vi "read_version.vi"() -> ()   [LabVIEW 2020]
uses:
  <vilib>/Automotive Diagnostic Command Set/Diagnostic Transport.llb/Transport Protocol Selector.ctl
  <vilib>/Automotive Diagnostic Command Set/Diagnostic Transport.llb/Property ID.ctl
  <vilib>/addons/Automotive Diagnostic Command Set/NI_Automotive Diagnostic Command Set.lvlib
panel:
  out "Response":u8[](array[numeric]) format="%.0x"
  out "CAN_log":string[][](table)
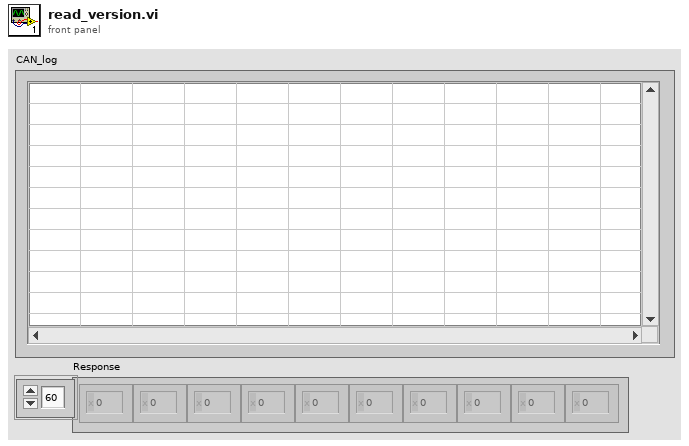
[diagram p1: front panel]
types:
  T1 = typedef "NI_Automotive Diagnostic Command Set.lvlib/Transport Protocol Selector.ctl" = enum16{"ISO TP - Normal Mode", "ISO TP - Mixed Mode", "VW TP 2.0", "Diagnostics on IP", "ISO TP LIN"}
  T2 = typedef "NI_Automotive Diagnostic Command Set.lvlib/Diag Reference.ctl" = cluster{"Diag CAN Handle":u32, "Transport Protocol":T1, "Receive Address Extension":u8, "Transmit Address Extension":u8, "Receive CAN Id":u32, "Transmit CAN Id":u32, "Log Frames ?":bool, "My TP Address":u8, "Other TP Address":u8, "T1":u16, "T2":u16, "T3":u16, "T4":u16, "Tx SN":u8, "Block Size":u8, "Rx SN":u8, "VW TP Initialized?":bool, "Tx block no":u8, "baud rate":u64, "Interface":string, "Channel Diag CAN Handle":u32, "UDP Connection ID":refnum<k16>, "TCP Connection ID":refnum<k5>, "Target IP Addr":u32, "Source Address":u16, "Target Address":u16, "Send Header NACK?":bool, "DLL Handle":u32, "NAD":u8, "Time Stamp read first":dbl, "Time Stamp read last":dbl, "Time Stamp write first":dbl, "Time Stamp write last":dbl, "Time Stamp write":dbl, "Time Stamp read":dbl, " I/O Mode":u32, "FD Baudrate":u64, "TX_DL":u16, "RX_DL":u16, "DoIP Protocol Version":T3, " Selected I/O Mode":u32, "TesterPresent Counter":u32, "TesterPresent Limit":u32, "TesterPresent Tick[ms]":i32, "TesterPresent RequireResponse?":bool, "TesterPresent Stored Ref?":bool, "TesterPresent Message":u8[], "TesterPresent Task Handle":i32, "TesterPresent Semaphore":T4, "Response Plausibility Check":u32, "Default Version?":bool, "Diagostic Globals":T5, "Session-based Properties?":bool}
  T3 = typedef "NI_Automotive Diagnostic Command Set.lvlib/DoIP Protocol Version.ctl" = u8
  T4 = typedef "Semaphore RefNum" = refnum<k1>
  T5 = typedef "NI_Automotive Diagnostic Command Set.lvlib/Diag Globals.ctl" = cluster{"Timeout FC (Bs)":u32, "Timeout CF (Cr)":u32, "Timeout Diag Command":u32, "Receive Block Size (BS)":u8, "Wait Time CF (STmin)":u8, "Max Waits (N_WFTmax)":u8, "Waits to Send (N_WAIT)":i32, "Time between Waits (TW)":u32, "Fill CAN Frames?":bool, "Fill Byte":u32, "Invalid Response as Error?":bool, "Max RspPending Count":u32, "VWTP Command Timeout":u32, "Transport Protocol":T1, "Diag CAN Handle":u32, "DLL Handle":u32, "Timeout RspPending":u32}
  T6 = typedef "NI_Automotive Diagnostic Command Set.lvlib/Property ID.ctl" = enum16{"Timeout Diag Command", "Timeout FC (Bs)", "Timeout CF (Cr)", "Receive Block Size (BS)", "Wait Time CF (STmin)", "Max Wait Frames (N_WFTmax)", "Wait Frames to Send (N_WAIT)", "Time between Waits (T_W)", "Fill CAN Frames", "Fill Byte", "Invalid Response as Error", "Max RspPending Count", "VWTP Command Timeout", "STmin", "P2min", "Termination", "Timeout RspPending", "LIN Sleep", "Actual CAN IO Mode", "Response Plausibility Check", "Session-based Properties"}
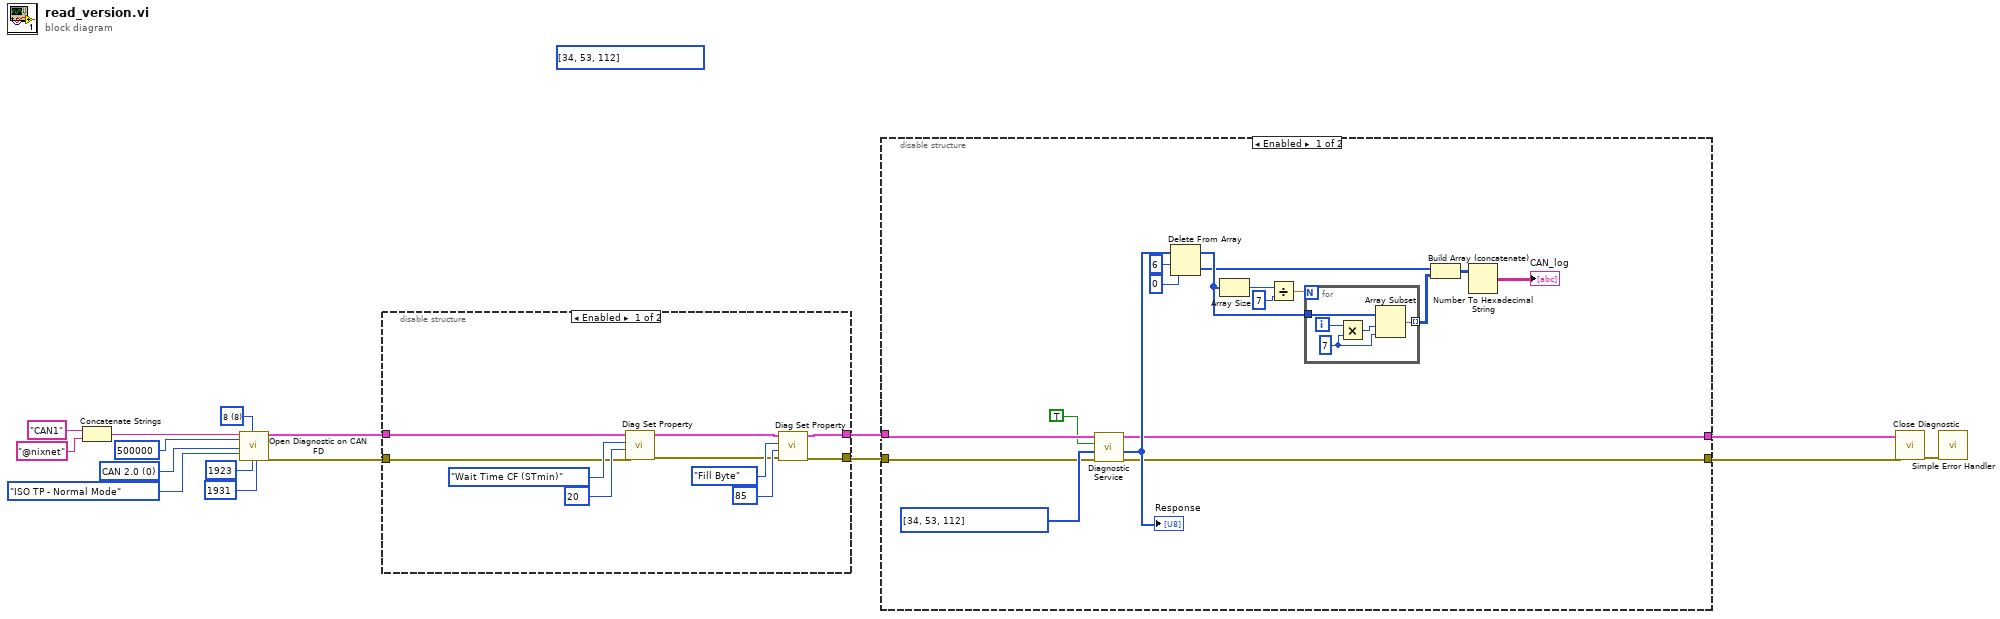
[diagram p0: block diagram]
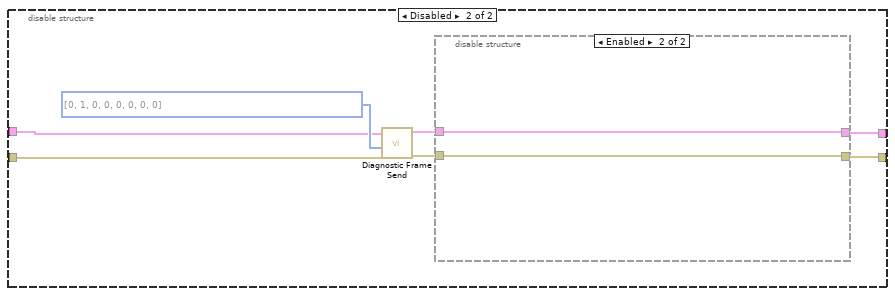
[diagram p3: hidden frame]
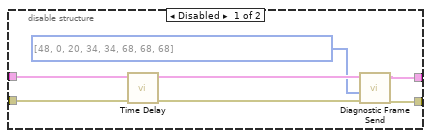
[diagram p4: hidden frame]
diagram:
  (unwired) u8[] [34, 53, 112] ("Request")
  w12 = u16 8 items=["8"=8, "12"=12, "16"=16, "20"=20, "24"=24, "32"=32, "48"=48, "64"=64] ("Max DLC")
  w14 = u32 0 items=["CAN 2.0", "CAN FD", "CAN FD+BRS", "ECU Determined"] ("IO Mode")
  n1 = Concatenate Strings("CAN1" ("Name"), "@nixnet") -> (w16:string)
  n2 = call <vilib>:"Open Diagnostic on CAN FD.vi"("CAN Interface"=w16, "Baud Rate"=u64 500000, "IO Mode"=w14, "Transport Protocol"=Transport_Protocol_Selector."ISO TP - Normal Mode", "Max DLC"=w12, "Transmit ID"=u32 1923, "Receive ID"=u32 1931) -> ("diag ref out"=w2:T2, "error out"=w1:errorcluster)  [unwired: 11 in]
  n3 = disable-structure shown="Enabled" {
    disable-tunnel: [w25 w28] -> w4
    disable-tunnel: [w24 w27] -> w3
    disable-tunnel: w2 -> [w20 w28]
    disable-tunnel: w1 -> [w18 w27]
    frame Enabled {
      n4 = call <vilib>:"Diag Set Property.vi"("error in (no error)"=w18, "property value"=u32 20, "property ID"=Property_ID."Wait Time CF (STmin)", "diag ref in"=w20) -> ("error out"=w17:errorcluster, "diag ref out"=w19:T2)  [unwired: 6 in]
      n5 = call <vilib>:"Diag Set Property.vi"("error in (no error)"=w17, "property value"=u32 85, "property ID"=Property_ID."Fill Byte", "diag ref in"=w19) -> ("error out"=w24:errorcluster, "diag ref out"=w25:T2)  [unwired: 6 in]
    }
    frame Disabled {
    }
  }
  n6 = disable-structure shown="Enabled" {
    disable-tunnel: w4 -> [w31 w52]
    disable-tunnel: w3 -> [w30 w51]
    disable-tunnel: [w34 w55] -> w6
    disable-tunnel: [w33 w54] -> w5
    frame Enabled {
      n7 = call <vilib>:"Diagnostic Service.vi"("error in (no error)"=w30, "data in"=u8[] [34, 53, 112] ("Request"), "require response?"=TRUE, "diag ref in"=w31) -> ("error out"=w33:errorcluster, "data out"=w45:u8[], "diag ref out"=w34:T2)  [unwired: 5 out]
      "Response" <- w45
      n8 = Delete From Array(array=w45, length=6, index=0) -> (deleted portion=w36:u8[], array with subset deleted=w39:u8[])
      n9 = Array Size(array=w39) -> (size(s)=w42:i32)
      n10 = Divide(x=w42, y=7) -> (x/y=w40:dbl)
      n11 = for {
        N: w40 -> [_]
        tunnel: w39 -> [w50]
        tunnel: [w46] -> w38 mode=indexing
        i -> [w48]
        w49 = 7 ("length")
        n12 = Multiply(x=w48, y=w49) -> (x*y=w47:i32)
        n13 = Array Subset(array=w50, index=w47, length=w49) -> (w46:u8[])
      }
      n14 = Build Array (concatenate)(w36, w38) -> (w37:u8[][])
      n15 = Number To Hexadecimal String(2:w37) -> (0:→"CAN_log":string[][])  [unwired: 1 in]
    }
    frame Disabled {
      n16 = call <vilib>:"Diagnostic Frame Send.vi"("error in (no error)"=w51, "data in"=u8[] [0, 1, 0, 0, 0, 0, 0, 0] ("Request"), "diag ref in"=w52) -> ("error out"=w57:errorcluster, "diag ref out"=w56:T2)  [unwired: 7 in]
      n17 = disable-structure shown="Enabled" {
        disable-tunnel: w57 -> [w63 w64]
        disable-tunnel: w56 -> [w62 w65]
        disable-tunnel: [w60 w65] -> w55
        disable-tunnel: [w59 w64] -> w54
        frame Disabled {
          n18 = call "Time Delay"("error in (no error)"=w63) -> ("error out"=w61:errorcluster)  [unwired: 10 in]
          n19 = call <vilib>:"Diagnostic Frame Send.vi"("error in (no error)"=w61, "data in"=u8[] [48, 0, 20, 34, 34, 68, 68, 68] ("Request"), "diag ref in"=w62) -> ("error out"=w59:errorcluster, "diag ref out"=w60:T2)  [unwired: 7 in]
        }
        frame Enabled {
        }
      }
    }
  }
  n20 = call <vilib>:"Close Diagnostic.vi"("error in (no error)"=w5, "diag ref in"=w6) -> ("error out"=w7:errorcluster)  [unwired: 9 out]
  n21 = call <vilib>:"Simple Error Handler.vi"("error in (no error)"=w7) -> ()  [unwired: 1 in, 8 out]
